vi "remove_control_shortcut_menu_item.vi"(8 "error in (no error)":errorcluster, 10 "Item Tag":string, 11 "IControlShortcutMenu In":refnum<class "IControlShortcutMenu.lvclass">) -> (0 "error out":errorcluster, 3 "IControlShortcutMenu Out":refnum<class "IControlShortcutMenu.lvclass">)   [LabVIEW 2015, in "ActorEvents.lvlib" / "IControlShortcutMenu.lvclass"]
uses:
  IControlShortcutMenu.lvclass
panel:
  # "STUB"
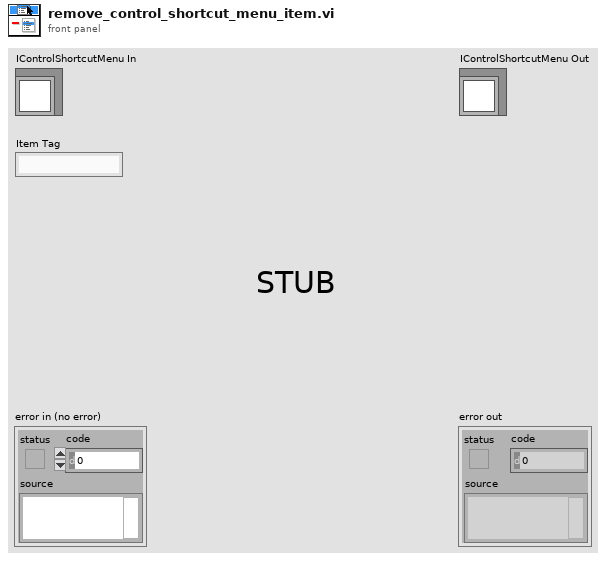
[diagram p1: front panel]
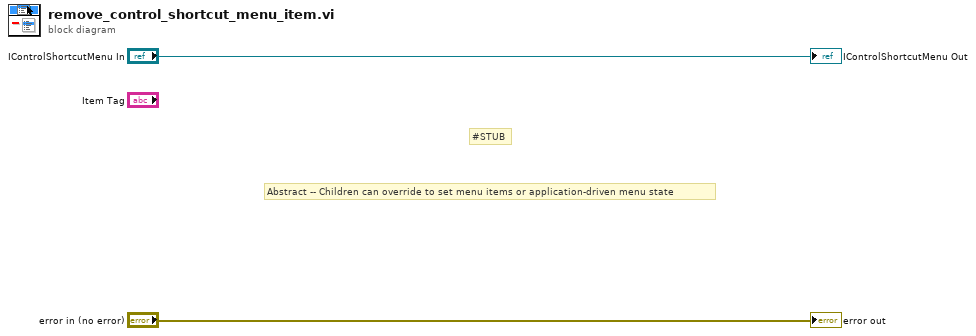
[diagram p0: block diagram]
diagram:
  # "#STUB"
  # "Abstract -- Children can override to set menu items or application-driven menu state"
  "error out" <- "error in (no error)"
  "IControlShortcutMenu Out" <- "IControlShortcutMenu In"
